vi "Base36 to Base10.vi"(1 "Base 36":string) -> (0 "Decimal":u64)   [LabVIEW 2016]
uses:
  Printing/Printing.lvlib
panel:
  out "Array 3":u64[](array[numeric])
  out "sum":u64
  out "x^y":ext
  out "Array":ext[](array[numeric]) format="%#_19g"
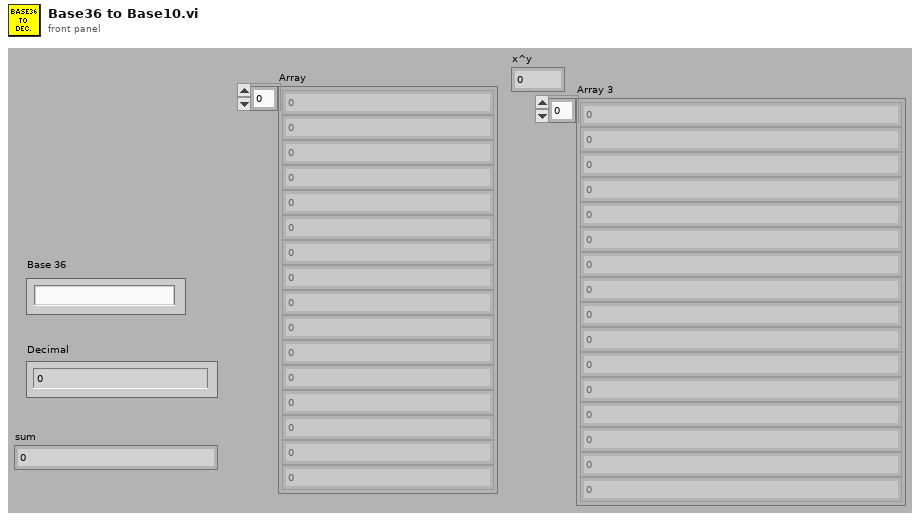
[diagram p1: front panel]
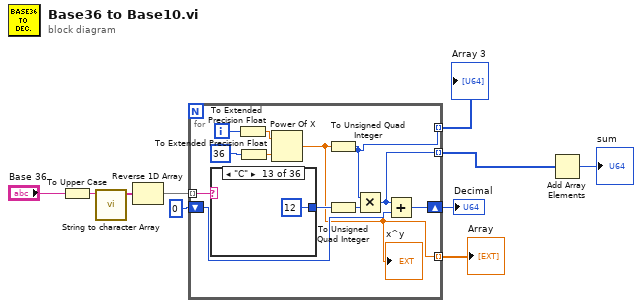
[diagram p0: block diagram]
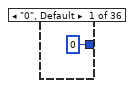
[diagram p2: hidden frame]
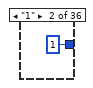
[diagram p3: hidden frame]
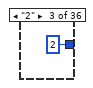
[diagram p4: hidden frame]
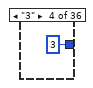
[diagram p5: hidden frame]
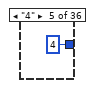
[diagram p6: hidden frame]
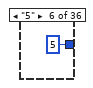
[diagram p7: hidden frame]
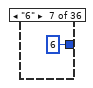
[diagram p8: hidden frame]
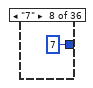
[diagram p9: hidden frame]
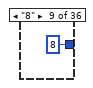
[diagram p10: hidden frame]
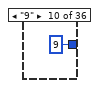
[diagram p11: hidden frame]
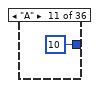
[diagram p12: hidden frame]
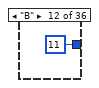
[diagram p13: hidden frame]
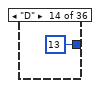
[diagram p14: hidden frame]
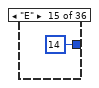
[diagram p15: hidden frame]
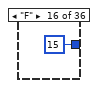
[diagram p16: hidden frame]
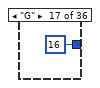
[diagram p17: hidden frame]
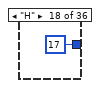
[diagram p18: hidden frame]
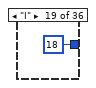
[diagram p19: hidden frame]
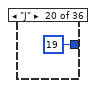
[diagram p20: hidden frame]
diagram:
  n1 = To Upper Case(1:"Base 36") -> (0:w6:string)
  n2 = call "String to character Array.vi"("String"=w6) -> ("Array"=w5:string[])  [unwired: 10 in]
  n3 = Reverse 1D Array(array=w5) -> (reversed array=w4:string[])
  n4 = for {
    shift-right: [w13] -> w9
    shift-left: u64 0 -> [w20]
    tunnel: [w19] -> w7 mode=indexing
    tunnel: w4 -> [w15] mode=indexing
    tunnel: [w12] -> w3 mode=indexing
    tunnel: [w11] -> w1 mode=indexing
    i -> [w14]
    n5 = case shown="\"C\"" w15 {
      tunnel: [0 1 2 3 4 5 6 7 8 9 10 11 12 13 14 15 16 17 18 19 20 21 22 23 24 25 26 27 28 29 30 31 32 33 34 35] -> w22
      frame "0", Default {
      }
      frame "1" {
      }
      frame "2" {
      }
      frame "3" {
      }
      frame "4" {
      }
      frame "5" {
      }
      frame "6" {
      }
      frame "7" {
      }
      frame "8" {
      }
      frame "9" {
      }
      frame "A" {
      }
      frame "B" {
      }
      frame "C" {
      }
      frame "D" {
      }
      frame "E" {
      }
      frame "F" {
      }
      frame "G" {
      }
      frame "H" {
      }
      frame "I" {
      }
      frame "J" {
      }
      frame "K" {
      }
      frame "L" {
      }
      frame "M" {
      }
      frame "N" {
      }
      frame "O" {
      }
      frame "P" {
      }
      frame "Q" {
      }
      frame "R" {
      }
      frame "S" {
      }
      frame "T" {
      }
      frame "U" {
      }
      frame "V" {
      }
      frame "W" {
      }
      frame "X" {
      }
      frame "Y" {
      }
      frame "Z" {
      }
    }
    n6 = To Extended Precision Float(1:w14) -> (0:w18:ext)
    n7 = To Extended Precision Float(1:36 ("x")) -> (0:w16:ext)
    n8 = Power Of X(1:w16, 2:w18) -> (0:w19:ext)
    "x^y" <- w19
    n9 = To Unsigned Quad Integer(1:w19) -> (0:w11:u64)
    n10 = To Unsigned Quad Integer(1:w22) -> (0:w21:u64)
    n11 = Multiply(x=w11, y=w21) -> (x*y=w12:u64)
    n12 = Add(x=w12, y=w20) -> (x+y=w13:u64)
  }
  "Decimal" <- w9
  "Array" <- w7
  "Array 3" <- w1
  n13 = Add Array Elements(numeric array=w3) -> (sum=→"sum":u64)
